vi "Get Use Diff Tool.vi"(8 "error in (no error)":errorcluster) -> (0 "error out":errorcluster, 2 "Diff in Descriptions?":bool)   [LabVIEW 2020, in "UI Configuration Manager.lvclass"]
uses:
  UI Configuration Manager.lvclass
  Framework/Configuration Manager/Configuration Manager.lvclass
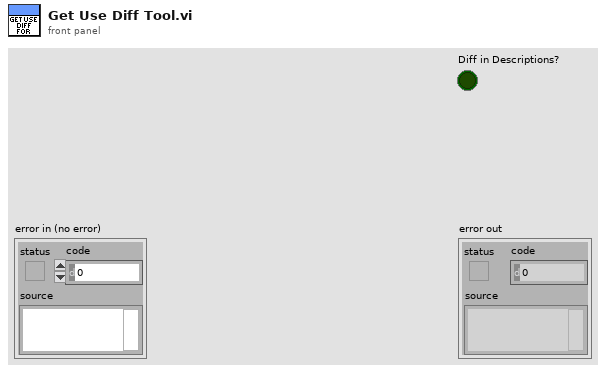
[diagram p1: front panel]
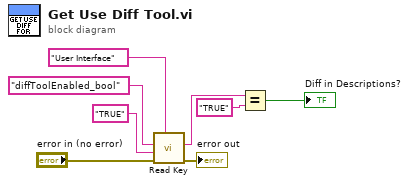
[diagram p0: block diagram]
diagram:
  n1 = call "Read Key.vi"("section"="User Interface", "error in (no error)"="error in (no error)", "default value"="TRUE", "key"="diffToolEnabled_bool") -> ("error out"=→"error out":errorcluster, "value"=w7:string)  [unwired: 6 in]
  n2 = Equal?(x=w7, y="TRUE" ("default value")) -> (x = y?=→"Diff in Descriptions?":bool)
